vi "GetPageProperty.vi"(8 "error in (no error)":errorcluster, 11 "This VI":refnum<vi>) -> (0 "error out":errorcluster, 1 "Settings":variant)   [LabVIEW 2019]
uses:
  Shared/Constants.vi
  Shared/SLSC EDS Shared.lvlib
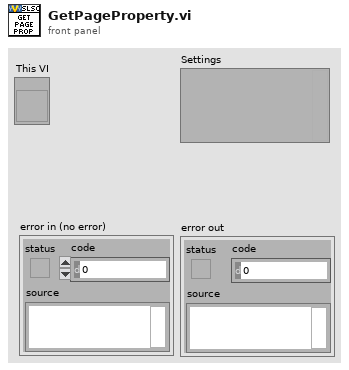
[diagram p1: front panel]
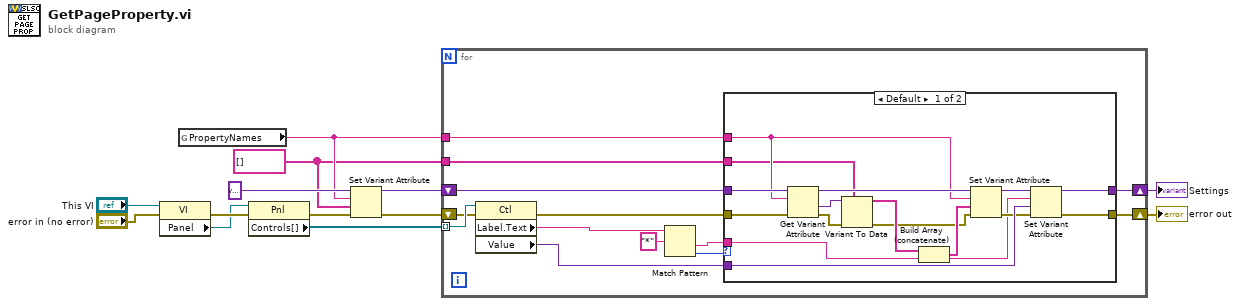
[diagram p0: block diagram]
diagram:
  w1 = string[] []
  n1 = property class="VI"(reference="This VI", error in="error in (no error)") -> (error out=w11:errorcluster, "Panel"=w10:refnum<vi>)  [unwired: 1 out]
  n2 = global read "Constants.vi" "PropertyNames"() -> (w4:string)
  n3 = property class="Pnl"(reference=w10, error in=w11) -> (error out=w3:errorcluster, "Controls[]"=w9:refnum<vi>[])  [unwired: 1 out]
  n4 = Set Variant Attribute(Variant=variant ("variant"), name=w4, value=w1, error in=w3) -> (Variant out=w5:variant, error out=w2:errorcluster)  [unwired: 1 out]
  n5 = for {
    tunnel: w9 -> [w26] mode=indexing
    shift-right: [w20] -> w8
    shift-left: w5 -> [w23]
    shift-right: [w19] -> w7
    shift-left: w2 -> [w25]
    tunnel: w4 -> [w17]
    tunnel: w1 -> [w14]
    n6 = property class="Ctl"(reference=w26, error in=w25) -> (error out=w21:errorcluster, "Label.Text"=w16:string, "Value"=w22:variant)  [unwired: 1 out]
    n7 = Match Pattern(string=w16, regular expression="*") -> (after substring=w18:string, offset past match=w15:i32)  [unwired: 1 in, 2 out]
    n8 = case shown="Default" w15 {
      tunnel: w18 -> [w32 _]
      tunnel: w23 -> [w39 w44]
      tunnel: w22 -> [w42 _]
      tunnel: w21 -> [w38 w43]
      tunnel: [w41 w44] -> w20
      tunnel: [w40 w43] -> w19
      tunnel: w17 -> [w34 _]
      tunnel: w14 -> [w30 _]
      frame Default {
        n9 = Get Variant Attribute(Variant=w39, name=w34, error in=w38) -> (duplicate Variant=w36:variant, value=w31:variant, error out=w28:errorcluster)  [unwired: 1 in, 1 out]
        n10 = Variant To Data(error in=w28, type=w30, Variant=w31) -> (data=w29:string[], error out=w27:errorcluster)
        n11 = Build Array (concatenate)(w29, w32) -> (w37:string[])
        n12 = Set Variant Attribute(Variant=w36, name=w34, value=w37, error in=w27) -> (Variant out=w35:variant, error out=w33:errorcluster)  [unwired: 1 out]
        n13 = Set Variant Attribute(Variant=w35, name=w32, value=w42, error in=w33) -> (Variant out=w41:variant, error out=w40:errorcluster)  [unwired: 1 out]
      }
      frame -1 {
      }
    }
  }
  "Settings" <- w8
  "error out" <- w7
